vi "ReadTubeCorrnFile.vi"(11 "PathToFile":path) -> (2 "F-CompArray":dbl[][](array[numeric]))   [LabVIEW 2012]
panel:
  out "FileContents":string
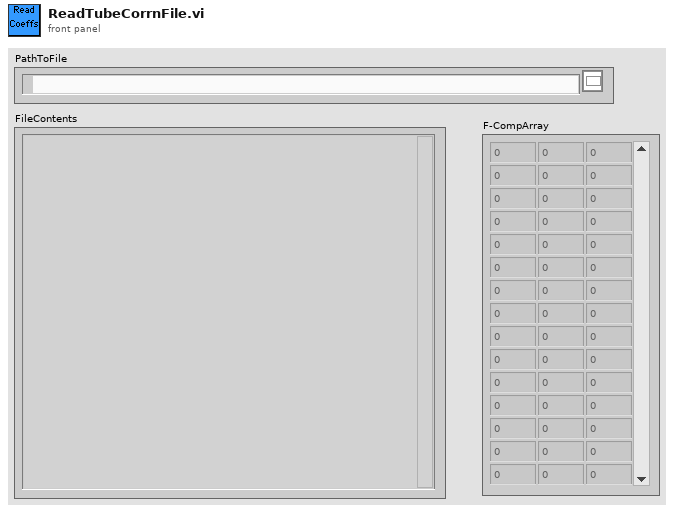
[diagram p1: front panel]
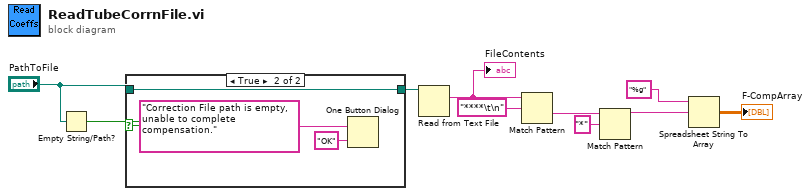
[diagram p0: block diagram]
diagram:
  n1 = Empty String/Path?(string/path="PathToFile") -> (empty?=w3:bool)
  n2 = case shown="True" w3 {
    tunnel: "PathToFile" -> [w11 w14]
    tunnel: [w11 w14] -> w1
    frame False {
    }
    frame True {
      n3 = One Button Dialog(message="Correction File path is empty, unable to complete compensation.", button name ("OK")="OK") -> ()  [unwired: 1 out]
    }
  }
  n4 = Read from Text File(file (use dialog)=w1) -> (text=w10:string)  [unwired: 3 in, 3 out]
  "FileContents" <- w10
  n5 = Match Pattern(string=w10, regular expression="****\t\n") -> (after substring=w6:string)  [unwired: 1 in, 3 out]
  n6 = Match Pattern(string=w6, regular expression="*") -> (before substring=w4:string)  [unwired: 1 in, 3 out]
  n7 = Spreadsheet String To Array(format string="%g", spreadsheet string=w4) -> (array=→"F-CompArray":dbl[][])  [unwired: 2 in]
